vi "SetDigitalPWMCommand.vi"(1 "Value":u8, 2 "Pin":u8) -> (0 "Command":T1)   [LabVIEW 2021]
uses:
  CommandType.ctl
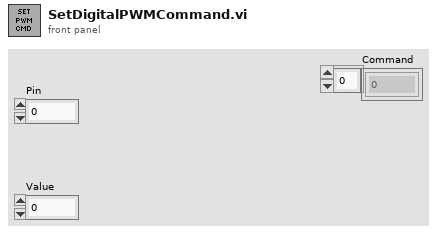
[diagram p1: front panel]
types:
  T1 = typedef "CommandType.ctl" = u8[]
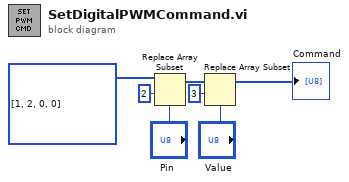
[diagram p0: block diagram]
diagram:
  n1 = Replace Array Subset(array=u8[] [1, 2, 0, 0], new element="Pin", index=2 ("indice")) -> (w4:u8[])
  n2 = Replace Array Subset(array=w4, new element="Value", index=3 ("indice")) -> (→"Command":u8[])
